vi "Store Configuration Parameters.vi"(8 "error in (no error)":errorcluster, 10 "refnum":T1, 11 "Example Configuration Dialog in":refnum<class "Slave Config.lvclass">) -> (0 "error out":errorcluster, 2 "refnum out":T1, 3 "Example Configuration Dialog out":refnum<class "Slave Config.lvclass">)   [LabVIEW 2016, in "Slave Config.lvclass"]
uses:
  <userlib>/Common Components/Slave Configuration/Slave Config.lvclass
  <vilib>/Utility/config.llb/Config Data RefNum.ctl
  <userlib>/Common Components/Slave Configuration/Slave Config.lvclass/Slave Config.ctl
  <userlib>/Configuration Dialog Actor/Configuration.lvclass
  <vilib>/Utility/config.llb/NI_LVConfig.lvlib
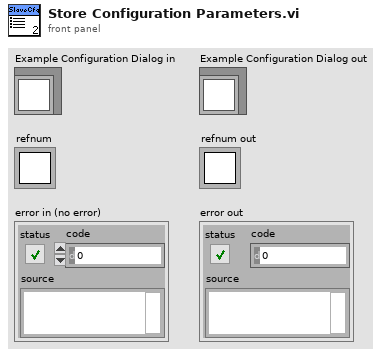
[diagram p1: front panel]
types:
  T1 = typedef "NI_LVConfig.lvlib/Config Data RefNum.ctl" = refnum<k1>
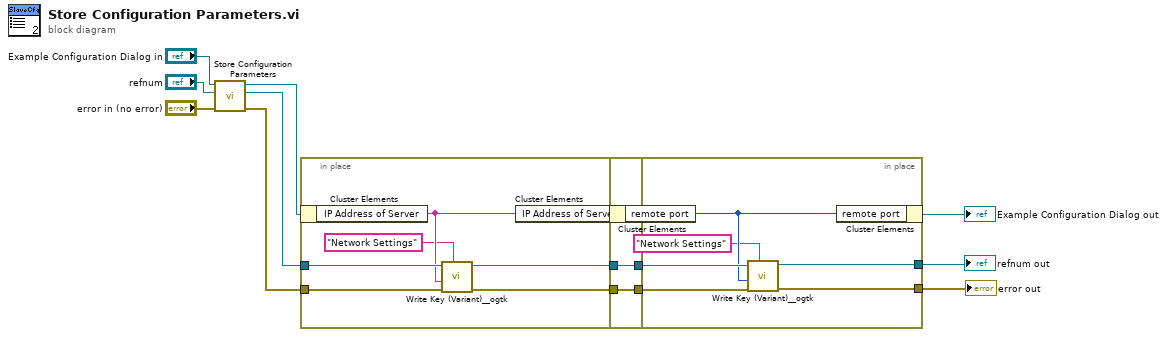
[diagram p0: block diagram]
diagram:
  n1 = call-parent "Store Configuration Parameters.vi"("error in (no error)"="error in (no error)", "refnum"="refnum", "Configuration in"="Example Configuration Dialog in") -> ("error out"=w3:errorcluster, "refnum out"=w5:T1, "Configuration out"=w9:refnum<class "Slave Config.lvclass">)  [unwired: 6 in]
  n2 = in-place "In Place Element Structure" {
    in-place-border: [w18] -> w6
    in-place-border: w5 -> [w17]
    in-place-border: w3 -> [w14]
    in-place-border: [w13] -> w2
    n3 = in-place-cluster #1(w9) -> ("IP Address of Server"=w16:string)
    n4 = call <userlib>:"Write Key (Variant)__ogtk.vi"("section"="Network Settings", "error in (no error)"=w14, "key-value"=w16, "refnum"=w17) -> ("error out"=w13:errorcluster, "refnum out"=w18:T1)  [unwired: 6 in]
    n5 = in-place-cluster #1("IP Address of Server"=w16) -> (w8:refnum<class "Slave Config.lvclass">)
  }
  n6 = in-place "In Place Element Structure" {
    in-place-border: w6 -> [w24]
    in-place-border: [w23] -> w4
    in-place-border: w2 -> [w20]
    in-place-border: [w19] -> w1
    n7 = in-place-cluster #2(w8) -> ("remote port"=w22:u16)
    n8 = call <userlib>:"Write Key (Variant)__ogtk.vi"("section"="Network Settings", "error in (no error)"=w20, "key-value"=w22, "refnum"=w24) -> ("error out"=w19:errorcluster, "refnum out"=w23:T1)  [unwired: 6 in]
    n9 = in-place-cluster #2("remote port"=w22) -> (→"Example Configuration Dialog out":refnum<class "Slave Config.lvclass">)
  }
  "error out" <- w1
  "refnum out" <- w4
